vi "FTS Set Acquisition Option Auto Gain.vi"(8 "error in (no error)":errorcluster, 10 "autoGain":bool, 11 "specIndex":u16) -> (0 "error out":errorcluster, 3 "function return":i32)   [LabVIEW 2010, in "FTSLib.lvlib"]
doc: "int __cdecl FTS_SetAcquisitionOption_AutoGain(unsigned short specIndex, bool autoGain);"
uses:
  FTSLib.lvlib
  FTSLib.dll
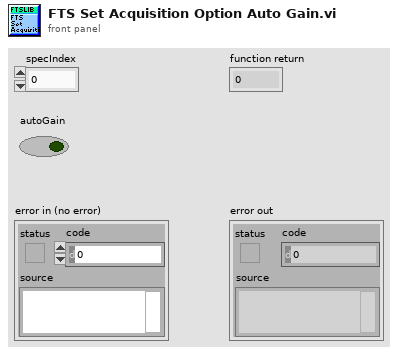
[diagram p1: front panel]
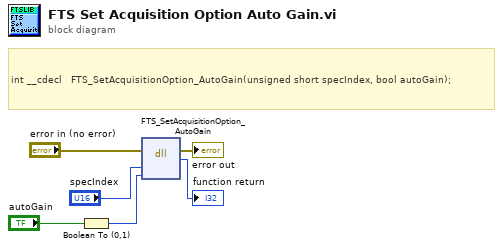
[diagram p0: block diagram]
diagram:
  # "int __cdecl   FTS_SetAcquisitionOption_AutoGain(unsigned short specIndex, bool autoGain);"
  n1 = Boolean To (0,1)(Boolean="autoGain") -> (0, 1=w3:i16)
  n2 = dll-call lib="FTSLib.*" fn="FTS_SetAcquisitionOption_AutoGain"(error in="error in (no error)", "specIndex"="specIndex", "autoGain"=w3) -> (error out=→"error out":errorcluster, →"function return":i32)  [unwired: 4 in, 1 out]
